vi "Fix test names.vi"() -> ()   [LabVIEW 2023]
uses:
  <vilib>/Utility/file.llb/Read Delimited Spreadsheet (string).vi
  <vilib>/Utility/file.llb/Write Delimited Spreadsheet (string).vi
panel:
  out "all rows 2":string[][](array[string])
  out "all rows":string[][](array[string])
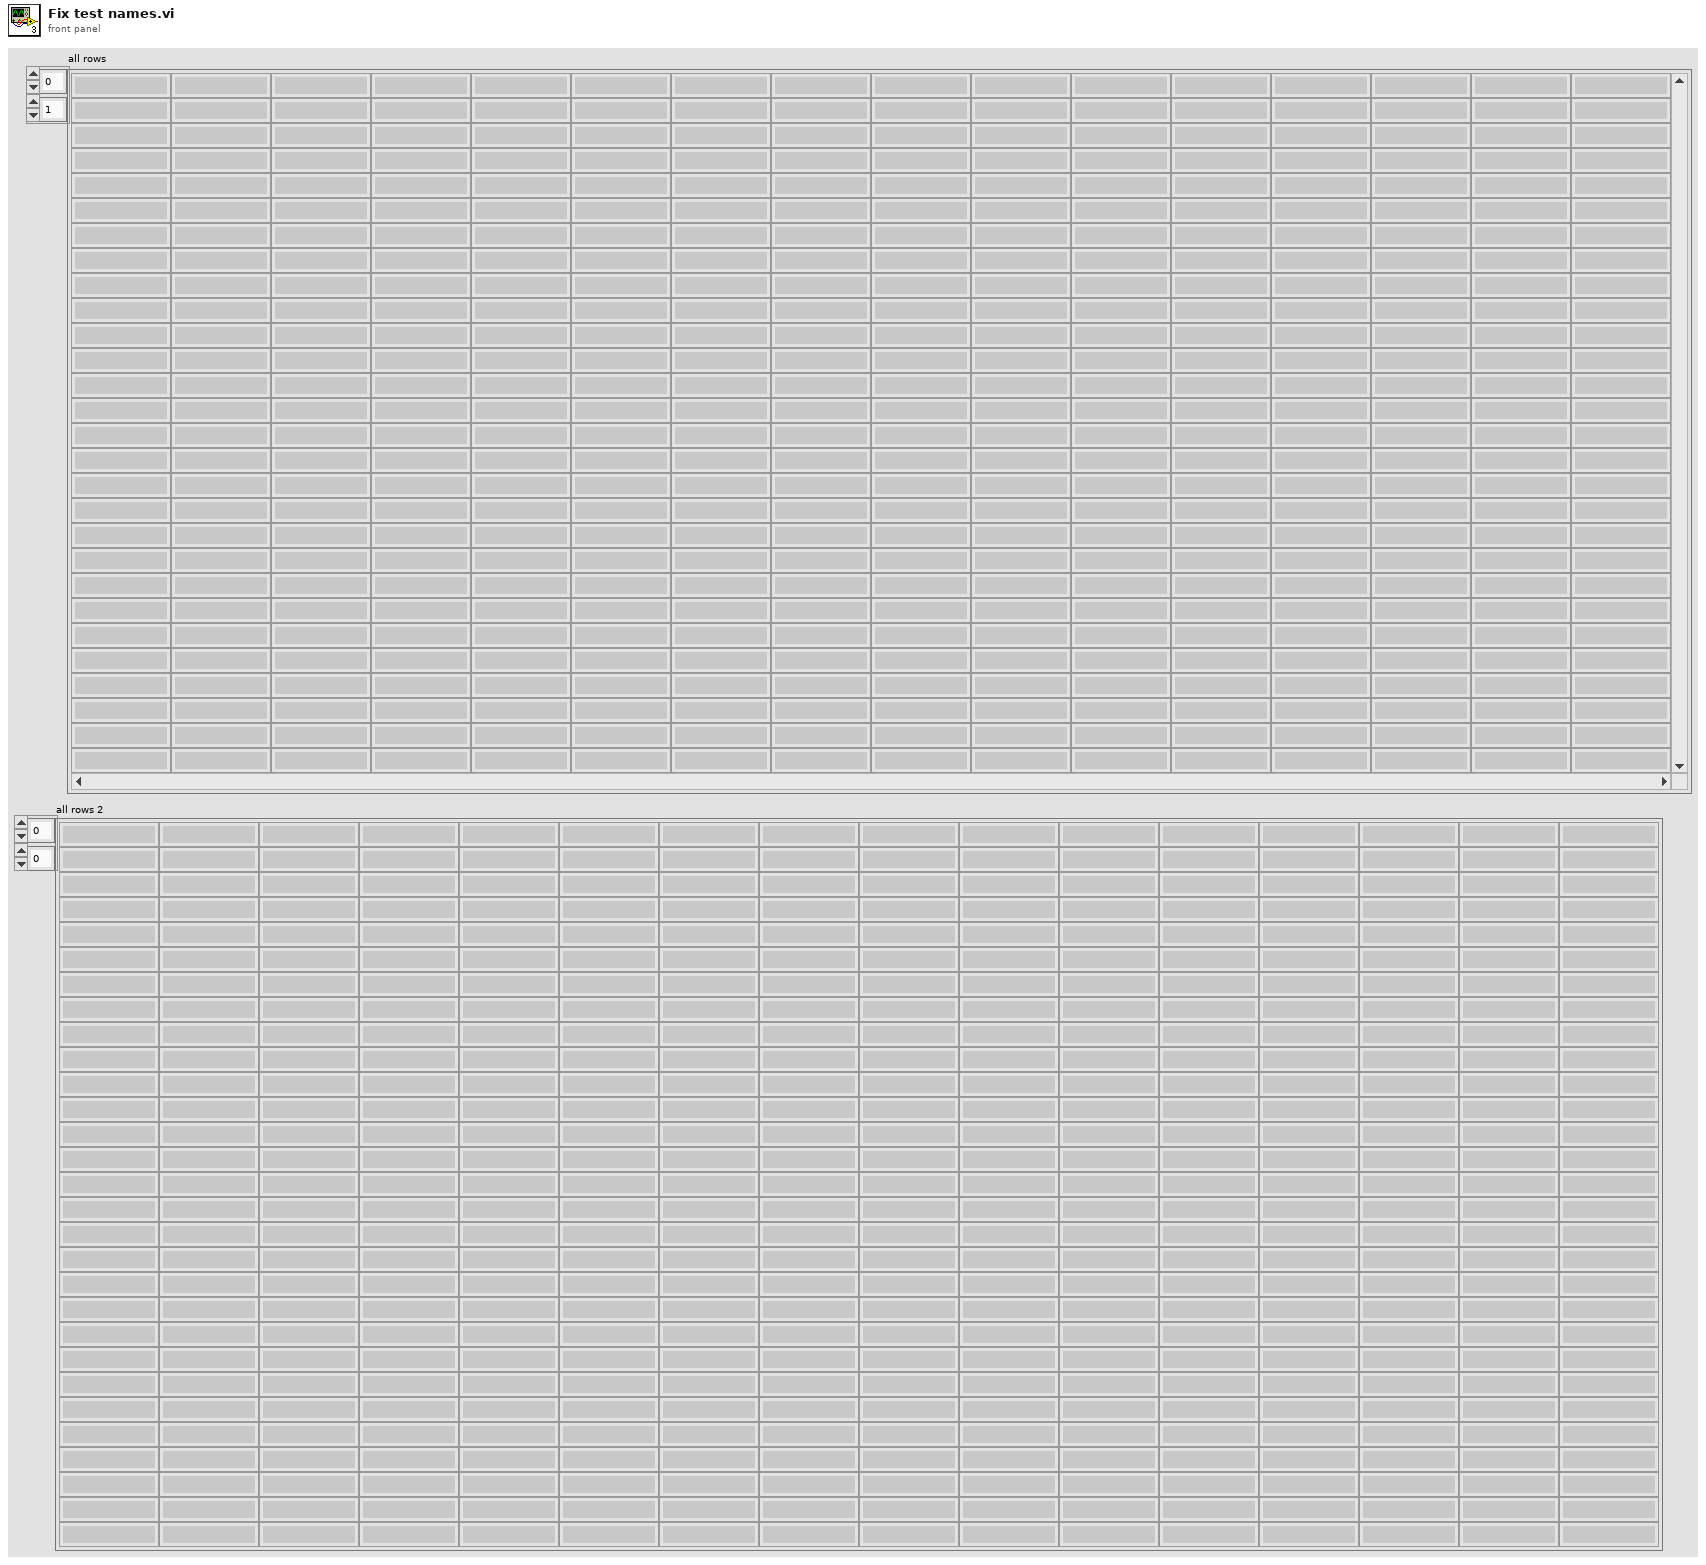
[diagram p1: front panel]
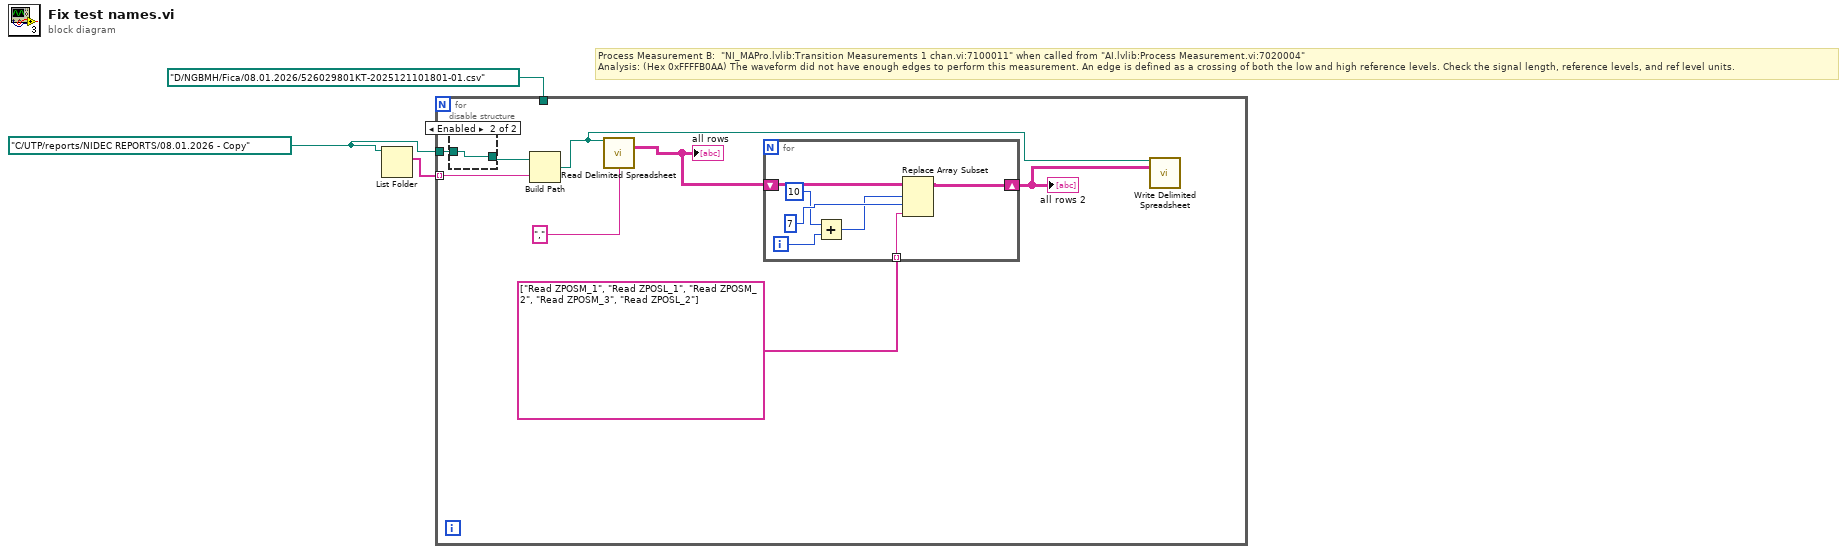
[diagram p0: block diagram]
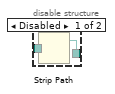
[diagram p2: hidden frame]
diagram:
  w2 = path "C:/UTP/reports/NIDEC REPORTS/08.01.2026 - Copy" ("path")
  # "Process Measurement B:  \"NI_MAPro.lvlib:Transition Measurements 1 chan.vi:7100011\" when called from \"AI.lvlib:Process Measurement.vi:7020004\" \nAnalysis: (Hex 0xFFFFB0AA) The waveform did not have enough edges to perform this measurement. An edge is defined as a crossing of both the low and high reference levels. Check the signal length, reference levels, and ref level units."
  n1 = List Folder(path=w2) -> (filenames=w1:string[])  [unwired: 3 in, 3 out]
  n2 = for {
    tunnel: path "D:/NGBMH/Fica/08.01.2026/526029801KT-2025121101801-01.csv" ("file path (dialog if empty)") -> [_]
    tunnel: w2 -> [w8]
    tunnel: w1 -> [w6] mode=indexing
    n3 = disable-structure shown="Enabled" {
      disable-tunnel: w8 -> [w13 w14]
      disable-tunnel: [w12 w14] -> w7
      frame Disabled {
        n4 = Strip Path(path=w13) -> (stripped path=w12:path)  [unwired: 1 out]
      }
      frame Enabled {
      }
    }
    n5 = Build Path(base path=w7, name or relative path=w6) -> (appended path=w5:path)
    n6 = call-poly <vilib>:"Read Delimited Spreadsheet.vi"("file path (dialog if empty)"=w5, "delimiter (\\t)"="," ("delimiter (\\t)")) -> ("all rows"=w10:string[][])  [unwired: 8 in, 5 out]
    "all rows" <- w10
    n7 = for {
      tunnel: string[] ["Read ZPOSM_1", "Read ZPOSL_1", "Read ZPOSM_2", "Read ZPOSM_3", "Read ZPOSL_2"] ("new element/subarray") -> [w19] mode=indexing
      shift-right: [w18] -> w4
      shift-left: w10 -> [w20]
      i -> [w21]
      n8 = Add(x=10 ("index (row)"), y=w21) -> (x+y=w15:i32)
      n9 = Replace Array Subset(array=w20, new element=w19, index (row)=w15, index (col)=7) -> (w18:string[][])
    }
    "all rows 2" <- w4
    n10 = call-poly <vilib>:"Write Delimited Spreadsheet.vi"("file path (dialog if empty)"=w5, "2D data"=w4) -> ()  [unwired: 12 in, 2 out]
  }
